vi "DMA Elements To Read.vi"(11 "Down Sample Divisor":i32) -> (3 "Num of Elements":u32)   [LabVIEW 2012]
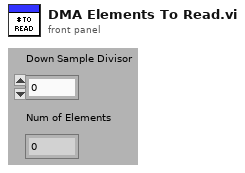
[diagram p1: front panel]
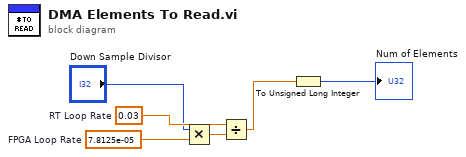
[diagram p0: block diagram]
diagram:
  w6 = 7.8125e-05  # FPGA Loop Rate
  w5 = 0.03  # RT Loop Rate
  n1 = Multiply(x="Down Sample Divisor", y=w6) -> (x*y=w4:dbl)
  n2 = Divide(x=w5, y=w4) -> (x/y=w1:dbl)
  n3 = To Unsigned Long Integer(number=w1) -> (unsigned 32bit integer=→"Num of Elements":u32)
